vi "make_stim_free_run.vi"(8 "error in":errorcluster, 10 "Device parameters":T1={"Triggered?"=FALSE, "Shutter channel"="", "Acquisition channels"="", "Acquisition sample rate"=1000.0, "Pixels to integrate"=100, "Effective sample rate"=0.0, "Read chunk size"=100, "Stimulation channel"="", "Stimulation sample rate"=1000.0} {"Pixels to integrate" min=1 max=100 step=1; "Read chunk size" min=100 max=100000; "Acquisition sample rate" min=10.0 max=10000.0 step=10.0; "Stimulation sample rate" min=10.0 max=10000.0}, 11 "Free run parameters":T2={"Stim onset"=5.0, "Stim frequency"=1.0, "Stim length"=0.001, "Sync shutter to acquisition"=TRUE} {"Stim length" min=0.001 max=0.1 step=0.01; "Stim onset" min=0.0 max=100.0; "Stim frequency" min=0.1 max=40.0 step=1.0}) -> (0 "error out":errorcluster, 2 "Stim array":dbl[](array[numeric]))   [LabVIEW 2010]
uses:
  typedefs/free_run_parameters.ctl
  typedefs/device_parameters.ctl
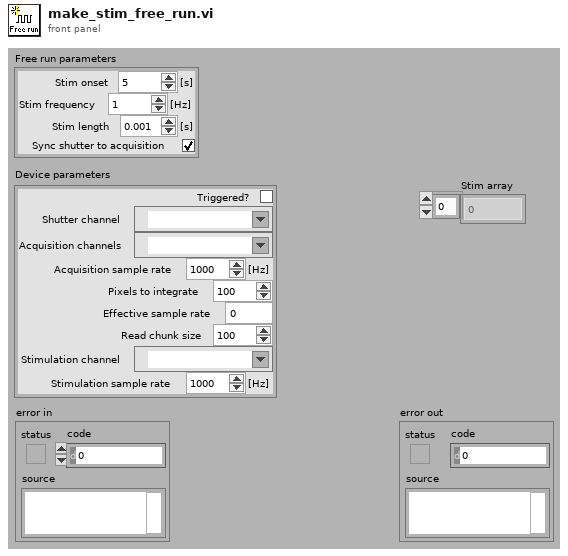
[diagram p1: front panel]
types:
  T1 = typedef "device_parameters.ctl" = cluster{"Triggered?":bool, "Shutter channel":tag, "Acquisition channels":tag, "Acquisition sample rate":dbl, "Pixels to integrate":i32, "Effective sample rate":dbl, "Read chunk size":i32, "Stimulation channel":tag, "Stimulation sample rate":dbl}
  T2 = typedef "free_run_parameters.ctl" = cluster{"Stim onset":dbl, "Stim frequency":dbl, "Stim length":dbl, "Sync shutter to acquisition":bool}
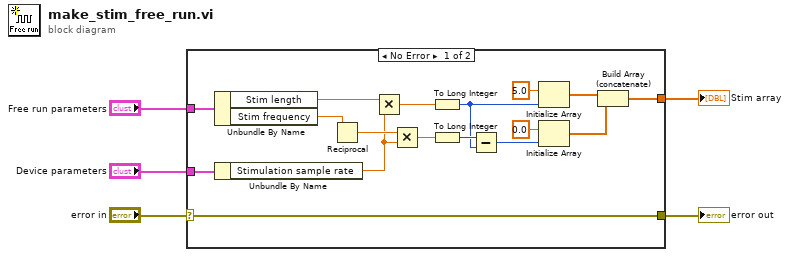
[diagram p0: block diagram]
diagram:
  n1 = case shown="No Error" "error in" {
    selector: "error in" -> [w22 w23]
    tunnel: [w22 w23] -> w4
    tunnel: "Free run parameters" -> [w20 _]
    tunnel: "Device parameters" -> [w21 _]
    tunnel: [w6 _] -> w1
    frame No Error {
      n2 = Unbundle By Name(w20) -> ("Stim length"=w18:dbl, "Stim frequency"=w16:dbl)
      n3 = Unbundle By Name(w21) -> ("Stimulation sample rate"=w14:dbl)
      n4 = Reciprocal(x=w16) -> (1/x=w15:dbl)
      n5 = Multiply(x=w18, y=w14) -> (x*y=w17:dbl)
      n6 = Multiply(x=w15, y=w14) -> (x*y=w13:dbl)
      n7 = To Long Integer(number=w17) -> (32bit integer=w11:i32)
      n8 = To Long Integer(number=w13) -> (32bit integer=w12:i32)
      n9 = Subtract(x=w12, y=w11) -> (x-y=w10:i32)
      n10 = Initialize Array(5.0 ("element"), w11) -> (w8:dbl[])
      n11 = Initialize Array(0.0 ("element"), w10) -> (w7:dbl[])
      n12 = Build Array (concatenate)(w8, w7) -> (w6:dbl[])
    }
    frame Error {
    }
  }
  "error out" <- w4
  "Stim array" <- w1
